vi "AlazarFFTBackgroundSubtractionSetRecordS16.vi"(3 "error in (no error)":errorcluster, 4 "Record":i16[](array[numeric]), 5 "DSP Handle":u64) -> (0 "error out":errorcluster, 1 "Return Code":u32, 2 "DSP Handle":u64)   [LabVIEW 2018]
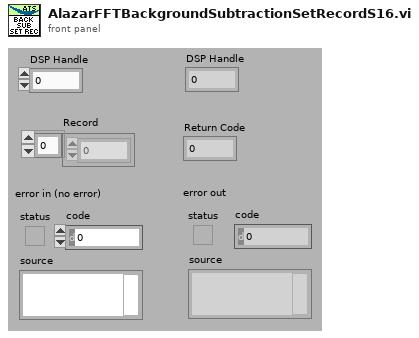
[diagram p1: front panel]
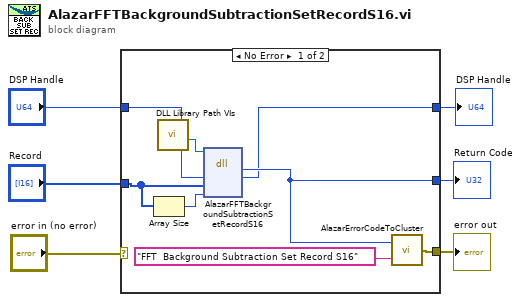
[diagram p0: block diagram]
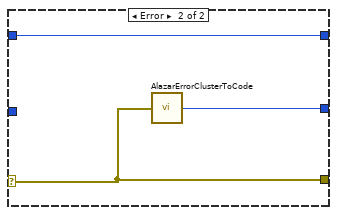
[diagram p2: hidden frame]
diagram:
  n1 = case shown="No Error" "error in (no error)" {
    selector: "error in (no error)" -> [_ w15]
    tunnel: [w11 w15] -> w5
    tunnel: [w13 w16] -> w1
    tunnel: "DSP Handle" -> [w14 w17]
    tunnel: [w10 w17] -> w3
    tunnel: "Record" -> [w9 _]
    frame No Error {
      n2 = Array Size(array=w9) -> (size(s)=w8:i32)
      n3 = call "DLL Library Path VIs.vi"() -> ("Alazar"=w7:path)  [unwired: 9 in, 2 out]
      n4 = dll-call lib="C:/Project/SerialSectOCT - FFT GPU/SerialSectOCT/Labview Software/DLL/ATSApi.dll" fn="AlazarFFTBackgroundSubtractionSetRecordS16"(path in=w7, "dspHandle"=w14, "record"=w9, "size_samples"=w8) -> ("return type"=w13:u32, "dspHandle"=w10:u64)  [unwired: 4 in, 2 out]
      n5 = call "AlazarErrorCodeToCluster.vi"("Message"="FFT  Background Subtraction Set Record S16", "Error Code"=w13) -> ("error out"=w11:errorcluster)
    }
    frame Error {
      n6 = call "AlazarErrorClusterToCode.vi"("error in (no error)"=w15) -> ("Error Code"=w16:u32)
    }
  }
  "DSP Handle" <- w3
  "error out" <- w5
  "Return Code" <- w1
